vi "Get Description.vi"(11 "Mocha in":refnum<class "Whip.lvclass">) -> (2 "Description":string, 3 "Mocha out":refnum<class "Whip.lvclass">)   [LabVIEW 2011, in "Whip.lvclass"]
uses:
  Whip.lvclass
  Whip.lvclass/Whip.ctl
  Beverage/Beverage.lvclass
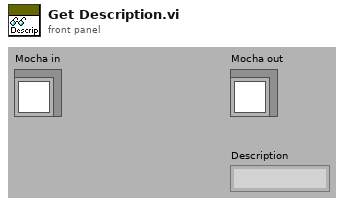
[diagram p1: front panel]
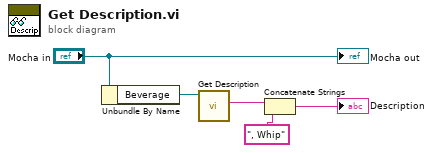
[diagram p0: block diagram]
diagram:
  n1 = Unbundle By Name("Mocha in") -> ("Beverage"=w4:refnum<class "Beverage.lvclass">)
  n2 = call-dynamic "Get Description.vi"("Beverage in"=w4) -> ("Description"=w3:string)  [unwired: 9 in, 1 out]
  n3 = Concatenate Strings(w3, ", Whip" ("string")) -> (→"Description":string)
  "Mocha out" <- "Mocha in"
